vi "FT10_Log Diff Volt TDMS Values.vi"(8 "error in (no error)":errorcluster, 9 "Log Cluster in":T2, 10 "Filename Cluster in":T1, 11 "Refnum in":T13) -> (0 "error out":errorcluster, 1 "Log Cluster out":T2, 2 "Filename Cluster out":T1, 3 "tdms file out":refnum<k34>)   [LabVIEW 2015]
doc: "Saves diff voltage to the TDMS file created when application started."
uses:
  Controls/Control_Log TDMS Filename.ctl
  Controls/Control_Log Cluster.ctl
  Controls/Control_Log Time.ctl
  Controls/Control_Log Waveform Cluster - Current.ctl
  Controls/Control_Log Analysis Cluster - Current.ctl
  Controls/Control_Log Activation Settings Cluster.ctl
  Controls/Control_Log Unitherm Load.ctl
  Controls/Control_Log Port.ctl
  Controls/Control_Log Mode.ctl
  Controls/Control_Log Power Level.ctl
  Controls/Control_Log Waveform Cluster - Diff Voltage.ctl
  Controls/Control_Log Analysis Cluster - Diff Voltage.ctl
  Controls/Control_Log Filename Cluster.ctl
  <vilib>/Waveform/WDTOps.llb/WDT Number of Waveform Samples DBL.vi
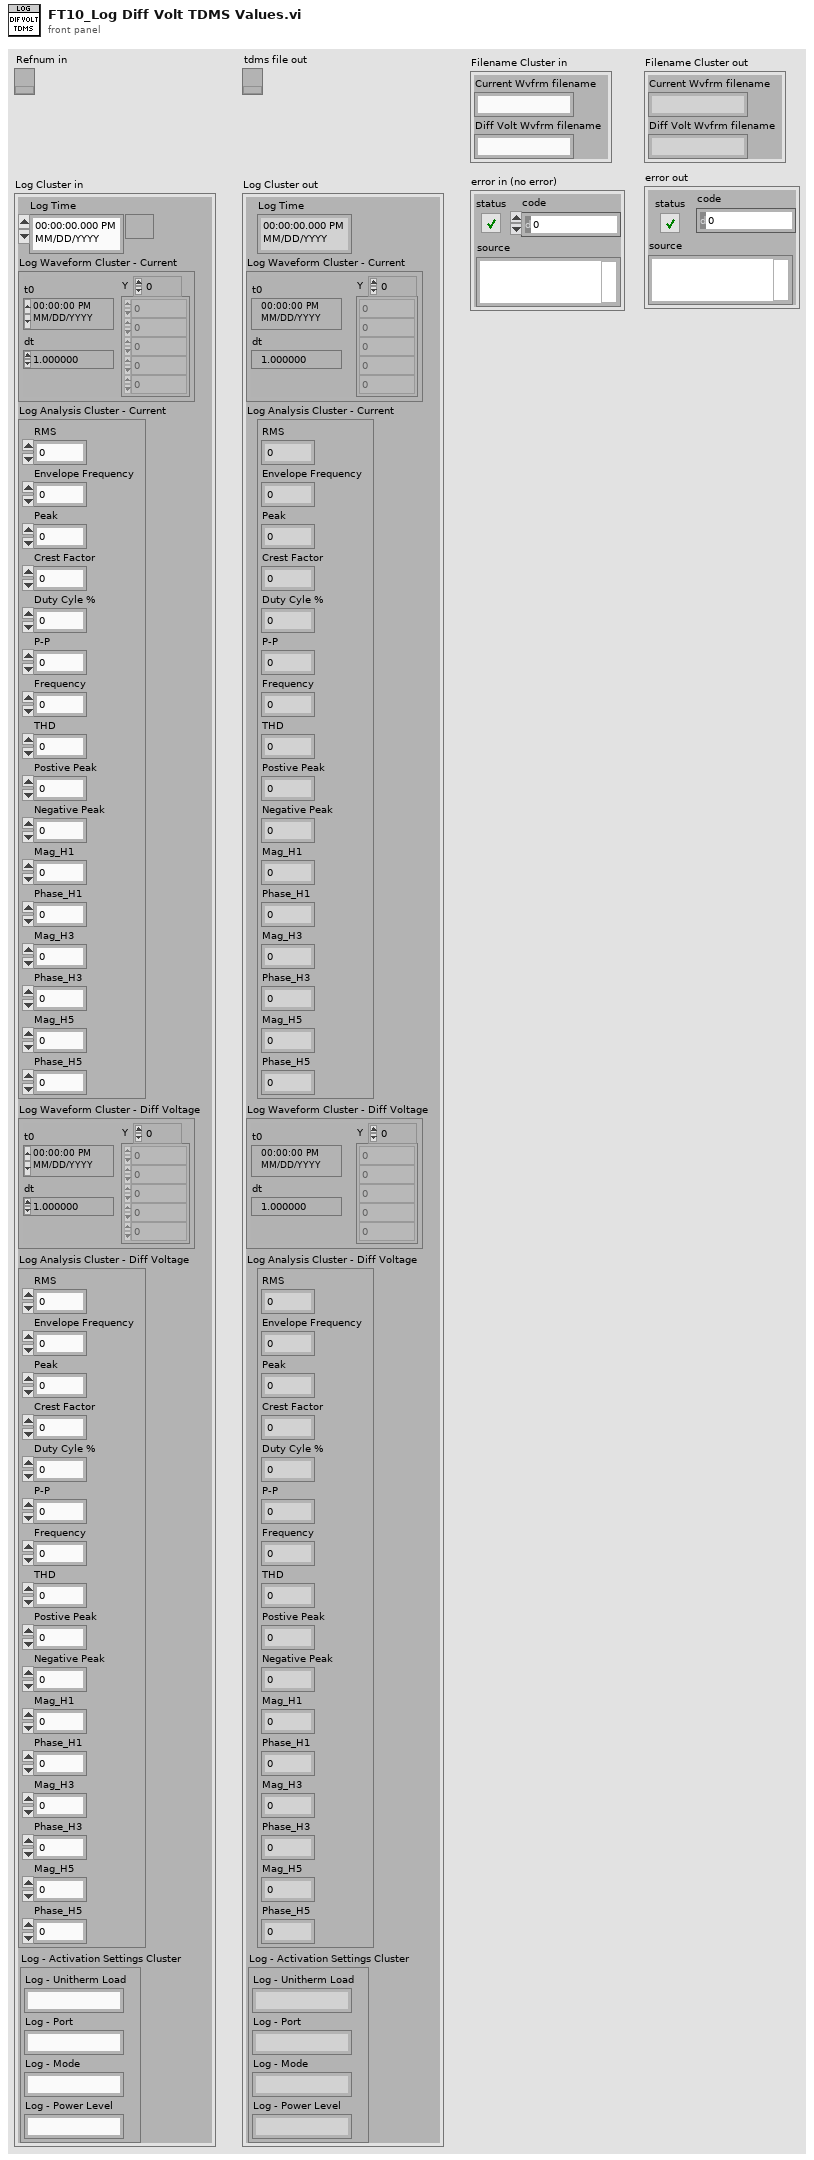
[diagram p1: front panel]
types:
  T1 = typedef "Control_Log Filename Cluster.ctl" = cluster{"Current Wvfrm filename":string, "Diff Volt Wvfrm filename":string}
  T2 = typedef "Control_Log Cluster.ctl" = cluster{"Log Time":T3, "Log Waveform Cluster - Current":T4, "Log Analysis Cluster - Current":T5, "Log - Activation Settings Cluster":T6, "Log Waveform Cluster - Diff Voltage":T11, "Log Analysis Cluster - Diff Voltage":T12}
  T3 = typedef "Control_Log Time.ctl" = timestamp
  T4 = typedef "Control_Log Waveform Cluster - Current.ctl" = waveform(dbl)
  T5 = typedef "Control_Log Analysis Cluster - Current.ctl" = cluster{"RMS":dbl, "Envelope Frequency":dbl, "Peak":dbl, "Crest Factor":dbl, "Duty Cyle %":dbl, "P-P":dbl, "Frequency":dbl, "THD":dbl, "Postive Peak":dbl, "Negative Peak":dbl, "Mag_H1":dbl, "Phase_H1":dbl, "Mag_H3":dbl, "Phase_H3":dbl, "Mag_H5":dbl, "Phase_H5":dbl}
  T6 = typedef "Control_Log Activation Settings Cluster.ctl" = cluster{"Log - Unitherm Load":T7, "Log - Port":T8, "Log - Mode":T9, "Log - Power Level":T10}
  T7 = typedef "Control_Log Unitherm Load.ctl" = string
  T8 = typedef "Control_Log Port.ctl" = string
  T9 = typedef "Control_Log Mode.ctl" = string
  T10 = typedef "Control_Log Power Level.ctl" = string
  T11 = typedef "Control_Log Waveform Cluster - Diff Voltage.ctl" = waveform(dbl)
  T12 = typedef "Control_Log Analysis Cluster - Diff Voltage.ctl" = cluster{"RMS":dbl, "Envelope Frequency":dbl, "Peak":dbl, "Crest Factor":dbl, "Duty Cyle %":dbl, "P-P":dbl, "Frequency":dbl, "THD":dbl, "Postive Peak":dbl, "Negative Peak":dbl, "Mag_H1":dbl, "Phase_H1":dbl, "Mag_H3":dbl, "Phase_H3":dbl, "Mag_H5":dbl, "Phase_H5":dbl}
  T13 = typedef "Control_Log TDMS Filename.ctl" = refnum<k34>
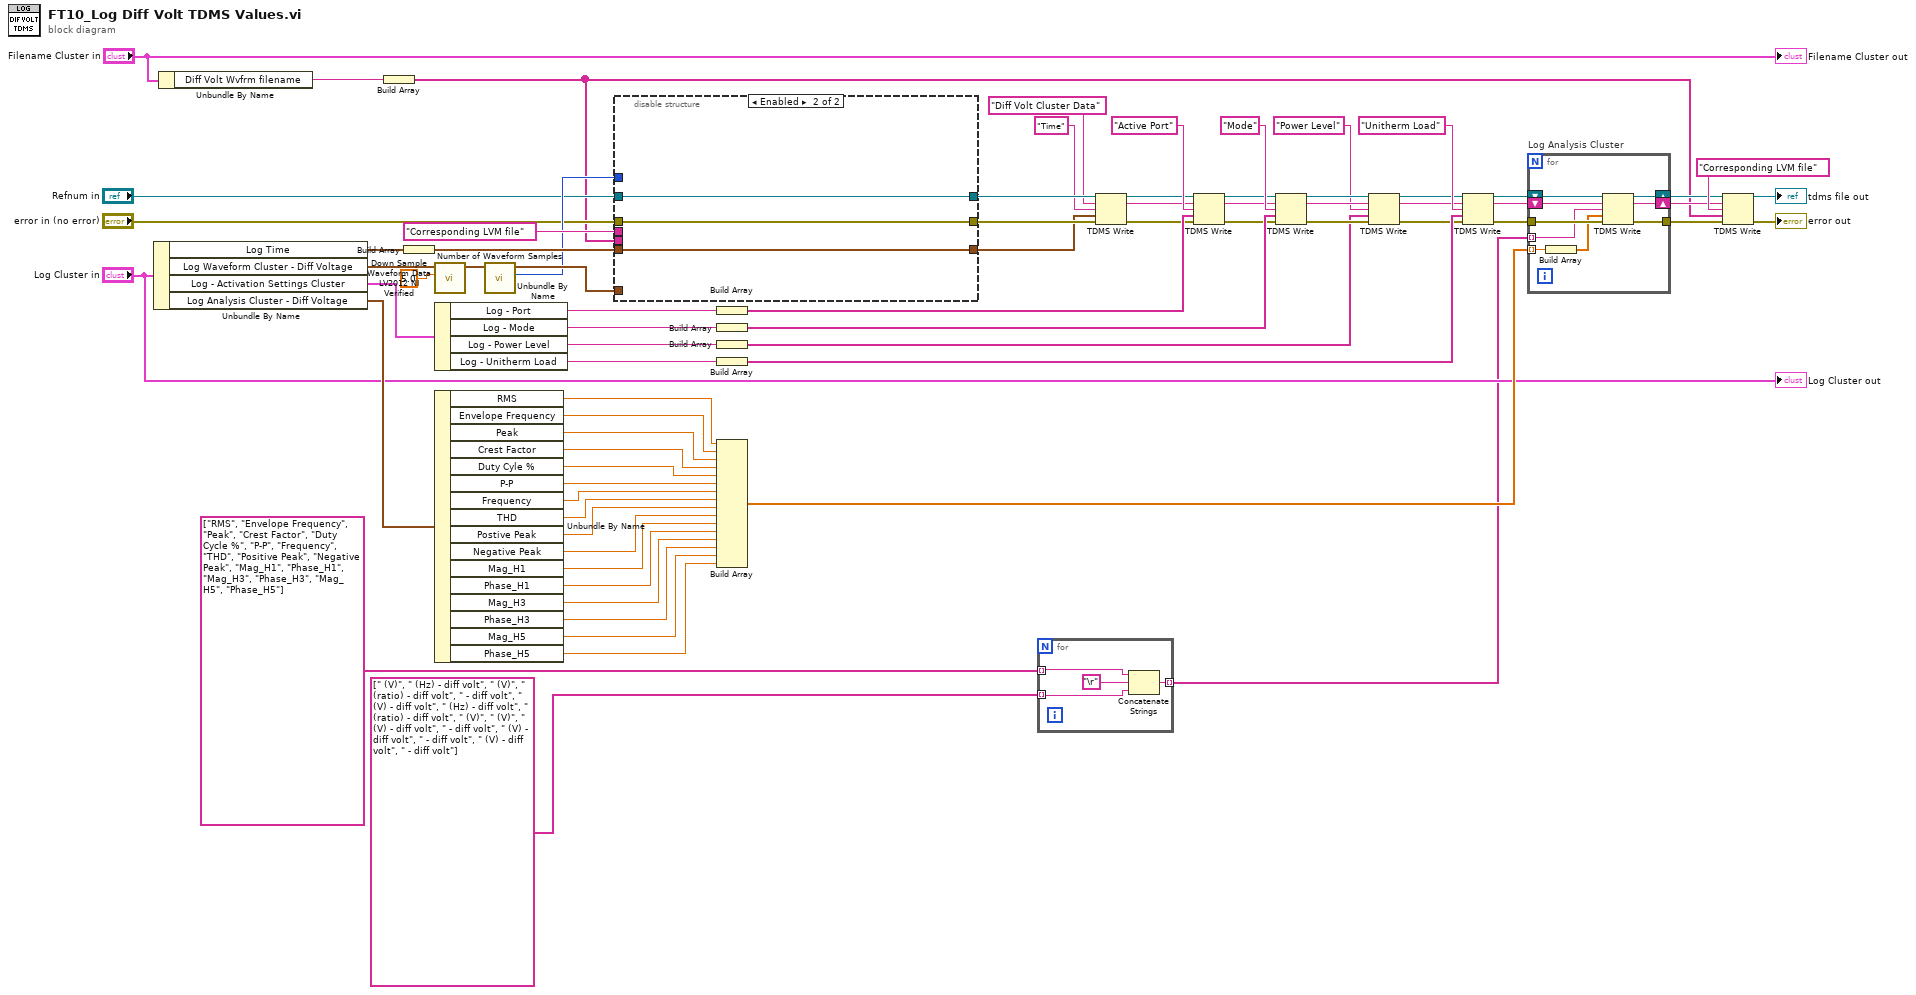
[diagram p0: block diagram]
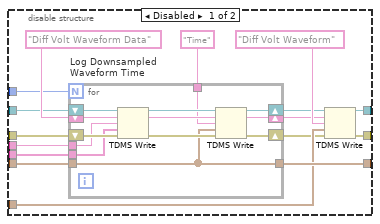
[diagram p2: hidden frame]
diagram:
  n1 = Unbundle By Name("Log Cluster in") -> ("Log Time"=w26:T3, "Log Waveform Cluster - Diff Voltage"=w20:T11, "Log - Activation Settings Cluster"=w66:T6, "Log Analysis Cluster - Diff Voltage"=w56:T12)
  n2 = Unbundle By Name("Filename Cluster in") -> ("Diff Volt Wvfrm filename"=w13:string)
  n3 = Build Array(w13) -> (w11:string[])
  n4 = Build Array(w26) -> (w27:T3[])
  n5 = call "Down Sample Waveform Data LV2012 NI Verified.vi"("Desired Sampling Rate"=5.0, "Waveform in"=w20) -> ("Waveform out"=w21:waveform(dbl))  [unwired: 8 in, 1 out]
  n6 = Unbundle By Name(w66) -> ("Log - Port"=w67:T8, "Log - Mode"=w69:T9, "Log - Power Level"=w71:T10, "Log - Unitherm Load"=w10:T7)
  n7 = Unbundle By Name(w56) -> ("RMS"=w32:dbl, "Envelope Frequency"=w33:dbl, "Peak"=w34:dbl, "Crest Factor"=w35:dbl, "Duty Cyle %"=w36:dbl, "P-P"=w37:dbl, "Frequency"=w38:dbl, "THD"=w39:dbl, "Postive Peak"=w40:dbl, "Negative Peak"=w41:dbl, "Mag_H1"=w42:dbl, "Phase_H1"=w43:dbl, "Mag_H3"=w44:dbl, "Phase_H3"=w45:dbl, "Mag_H5"=w46:dbl, "Phase_H5"=w47:dbl)
  n8 = call-poly <vilib>:"Number of Waveform Samples.vi"("waveform in"=w21) -> ("number of samples"=w24:i32, "waveform out"=w28:waveform(dbl))  [unwired: 8 in, 1 out]
  n9 = disable-structure shown="Enabled" {
    disable-tunnel: [w89 w105] -> w50
    disable-tunnel: [w88 w106] -> w49
    disable-tunnel: [w87 w104] -> w31
    disable-tunnel: w28 -> [w86 _]
    disable-tunnel: w27 -> [w81 w104]
    disable-tunnel: "Corresponding LVM file" ("channel name(s) in (Untitled)") -> [w80 _]
    disable-tunnel: w24 -> [w78 _]
    disable-tunnel: "Refnum in" -> [w77 w106]
    disable-tunnel: "error in (no error)" -> [w76 w105]
    disable-tunnel: w11 -> [w75 _]
    frame Disabled {
      n10 = for "Log Downsampled Waveform Time" {
        N: w78 -> [_]
        tunnel: w80 -> [w100]
        tunnel: w81 -> [w92]
        shift-right: [w97] -> w83
        shift-left: "Diff Volt Waveform Data" ("group name in (Untitled)") -> [w103]
        shift-right: [w98] -> w82
        shift-left: w77 -> [w102]
        shift-right: [w94] -> w84
        shift-left: w76 -> [w101]
        tunnel: [w92] -> w87
        tunnel: "Time" ("channel name(s) in (Untitled)") -> [w93]
        tunnel: w75 -> [w91]
        n11 = TDMS Write(0:w102, 5:w103, 7:w100, 9:w91, 11:w101) -> (4:w99:refnum<k34>, 6:w96:string, 15:w95:errorcluster)  [unwired: 1 in, 1 out]
        n12 = TDMS Write(0:w99, 5:w96, 7:w93, 9:w92, 11:w95) -> (4:w98:refnum<k34>, 6:w97:string, 15:w94:errorcluster)  [unwired: 1 in, 1 out]
      }
      n13 = TDMS Write(0:w82, 5:w83, 7:"Diff Volt Waveform" ("channel name(s) in (Untitled)"), 9:w86, 11:w84) -> (4:w88:refnum<k34>, 15:w89:errorcluster)  [unwired: 1 in, 2 out]
    }
    frame Enabled {
    }
  }
  n14 = Build Array(w67) -> (w68:T8[])
  n15 = Build Array(w69) -> (w70:T9[])
  n16 = Build Array(w71) -> (w1:T10[])
  n17 = Build Array(w10) -> (w9:T7[])
  n18 = Build Array(w32, w33, w34, w35, w36, w37, w38, w39, w40, w41, w42, w43, w44, w45, w46, w47) -> (w48:dbl[])
  n19 = for {
    tunnel: string[] ["RMS", "Envelope Frequency", "Peak", "Crest Factor", "Duty Cycle %", "P-P", "Frequency", "THD", "Positive Peak", "Negative Peak", "Mag_H1", "Phase_H1", "Mag_H3", "Phase_H3", "Mag_H5", "Phase_H5"] ("channel name(s) in (Untitled)") -> [w109] mode=indexing
    tunnel: string[] [" (V)", " (Hz) - diff volt", " (V)", " (ratio) - diff volt", " - diff volt", " (V) - diff volt", " (Hz) - diff volt", " (ratio) - diff volt", " (V)", " (V)", " (V) - diff volt", " - diff volt", " (V) - diff volt", " - diff volt", " (V) - diff volt", " - diff volt"] ("channel name(s) in (Untitled)") -> [w108] mode=indexing
    tunnel: [w107] -> w15 mode=indexing
    n20 = Concatenate Strings(w109, "\r", w108) -> (w107:string)
  }
  n21 = TDMS Write(0:w49, 5:"Diff Volt Cluster Data" ("group name in (Untitled)"), 7:"Time" ("channel name(s) in (Untitled)"), 9:w31, 11:w50) -> (4:w61:refnum<k34>, 6:w59:string, 15:w64:errorcluster)  [unwired: 1 in, 1 out]
  n22 = TDMS Write(0:w61, 5:w59, 7:"Active Port" ("channel name(s) in (Untitled)"), 9:w68, 11:w64) -> (4:w62:refnum<k34>, 6:w58:string, 15:w65:errorcluster)  [unwired: 1 in, 1 out]
  n23 = TDMS Write(0:w62, 5:w58, 7:"Mode" ("channel name(s) in (Untitled)"), 9:w70, 11:w65) -> (4:w8:refnum<k34>, 6:w7:string, 15:w6:errorcluster)  [unwired: 1 in, 1 out]
  n24 = TDMS Write(0:w8, 5:w7, 7:"Power Level" ("channel name(s) in (Untitled)"), 9:w1, 11:w6) -> (4:w5:refnum<k34>, 6:w4:string, 15:w3:errorcluster)  [unwired: 1 in, 1 out]
  n25 = TDMS Write(0:w5, 5:w4, 7:"Unitherm Load" ("channel name(s) in (Untitled)"), 9:w9, 11:w3) -> (4:w60:refnum<k34>, 6:w57:string, 15:w63:errorcluster)  [unwired: 1 in, 1 out]
  n26 = for "Log Analysis Cluster" {
    shift-right: [w118] -> w53
    shift-left: w60 -> [w119]
    shift-right: [w116] -> w54
    shift-left: w57 -> [w117]
    tunnel: w63 -> [w115]
    tunnel: [w114] -> w51
    tunnel: w48 -> [w113] mode=indexing
    tunnel: w15 -> [w111] mode=indexing
    n27 = Build Array(w113) -> (w112:dbl[])
    n28 = TDMS Write(0:w119, 5:w117, 7:w111, 9:w112, 11:w115) -> (4:w118:refnum<k34>, 6:w116:string, 15:w114:errorcluster)  [unwired: 1 in, 1 out]
  }
  n29 = TDMS Write(0:w53, 5:w54, 7:"Corresponding LVM file" ("channel name(s) in (Untitled)"), 9:w11, 11:w51) -> (4:→"tdms file out":refnum<k34>, 15:→"error out":errorcluster)  [unwired: 1 in, 2 out]
  "Log Cluster out" <- "Log Cluster in"
  "Filename Cluster out" <- "Filename Cluster in"
